vi "System Command.vi"(8 "error in (no error)":errorcluster, 11 "command":string) -> (0 "error out":errorcluster, 1 "return code":i32, 2 "standard error":string, 3 "standard output":string)   [LabVIEW 2019]
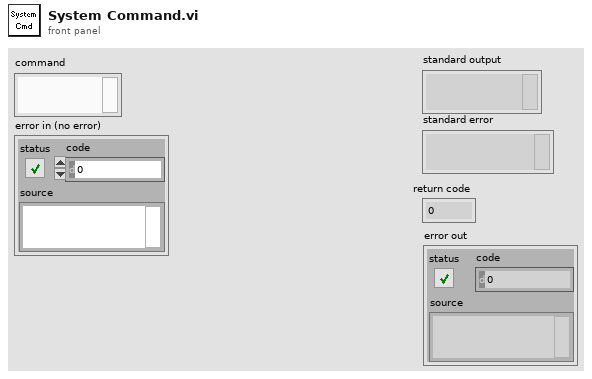
[diagram p1: front panel]
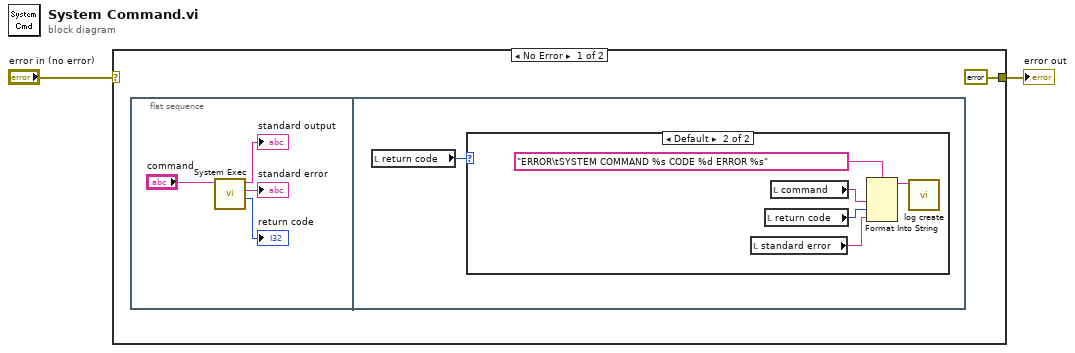
[diagram p0: block diagram]
diagram:
  n1 = case shown="No Error" "error in (no error)" {
    selector: "error in (no error)" -> [_ w14]
    tunnel: [errorcluster {"status"=FALSE, "code"=0, "source"=""} ("error IO") w14] -> w1
    frame No Error {
      n2 = flat-sequence {
        frame #0 {
          n3 = call <vilib>:"System Exec.vi"("command line"="command") -> ("return code"=→"return code":i32, "standard error"=→"standard error":string, "standard output"=→"standard output":string)  [unwired: 7 in, 1 out]
        }
        frame #1 {
          n4 = local read "return code"() -> (w8:i32)
          n5 = case shown="Default" w8 {
            frame 0 {
            }
            frame Default {
              n6 = local read "standard error"() -> (w11:string)
              n7 = local read "return code"() -> (w10:i32)
              n8 = local read "command"() -> (w9:string)
              n9 = Format Into String(format string="ERROR\tSYSTEM COMMAND %s CODE %d ERROR %s" ("message"), w9, w10, w11) -> (resulting string=w12:string)  [unwired: 2 in, 1 out]
              n10 = call "log create.vi"("message"=w12) -> ()  [unwired: 11 in]
            }
          }
        }
      }
    }
    frame Error {
    }
  }
  "error out" <- w1
